vi "_PC_MS_SubVI mathRoundTo.vi"(6 "Up/Down":bool, 7 "Digit":i32, 9 "Numeric":dbl) -> (1 "Round to":dbl)   [LabVIEW 2018]
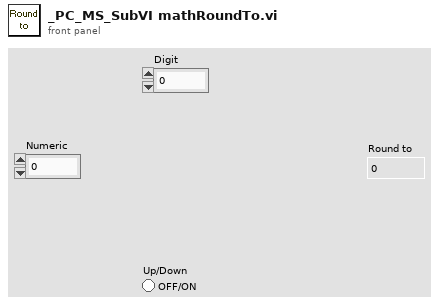
[diagram p1: front panel]
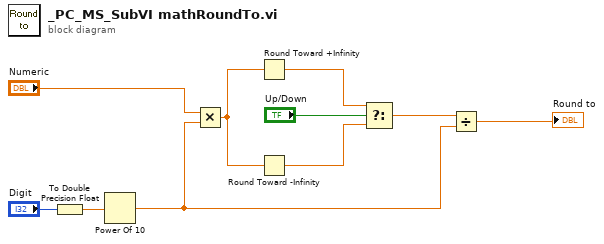
[diagram p0: block diagram]
diagram:
  n1 = To Double Precision Float(number="Digit") -> (double precision float=w2:dbl)
  n2 = Power Of 10(x=w2) -> (10^x=w3:dbl)
  n3 = Multiply(x="Numeric", y=w3) -> (x*y=w8:dbl)
  n4 = Round Toward +Infinity(x=w8) -> (ceil(x): smallest int >= x=w6:dbl)
  n5 = Round Toward -Infinity(1:w8) -> (0:w7:dbl)
  n6 = Select(t=w6, s="Up/Down", f=w7) -> (s? t:f=w5:dbl)
  n7 = Divide(x=w5, y=w3) -> (x/y=→"Round to":dbl)
